vi "Trim Channel Info.vi"(8 "error IO":errorcluster, 11 "Raw Channel Info":string[][](array[string])) -> (0 "error out":errorcluster, 3 "Trimmed Channel Info":T1[](array[typedef]))   [LabVIEW 2021, in "myRIOMetaDataObj.lvclass"]
uses:
  myRIOMetaDataObj.lvclass
  IODetail.ctl
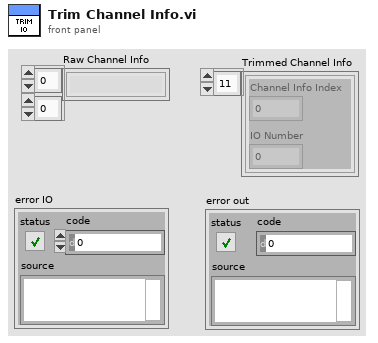
[diagram p1: front panel]
types:
  T1 = typedef "myRIOMetaDataObj.lvclass/IODetail.ctl" = cluster{"Channel Info Index":i8, "IO Number":i8}
  T2 = enum16{"Initial", "Get Channel Info Index by Name", "Get Channel Info by Index", "Get Channel Info by Img Index"}
  T3 = typedef "myRIOMetaDataObj.lvclass/ChannelInfo.ctl" = cluster{"Priority":u16, "Channel Shortcut":string, "Channel Description":string, "Channl Image Index":u16}
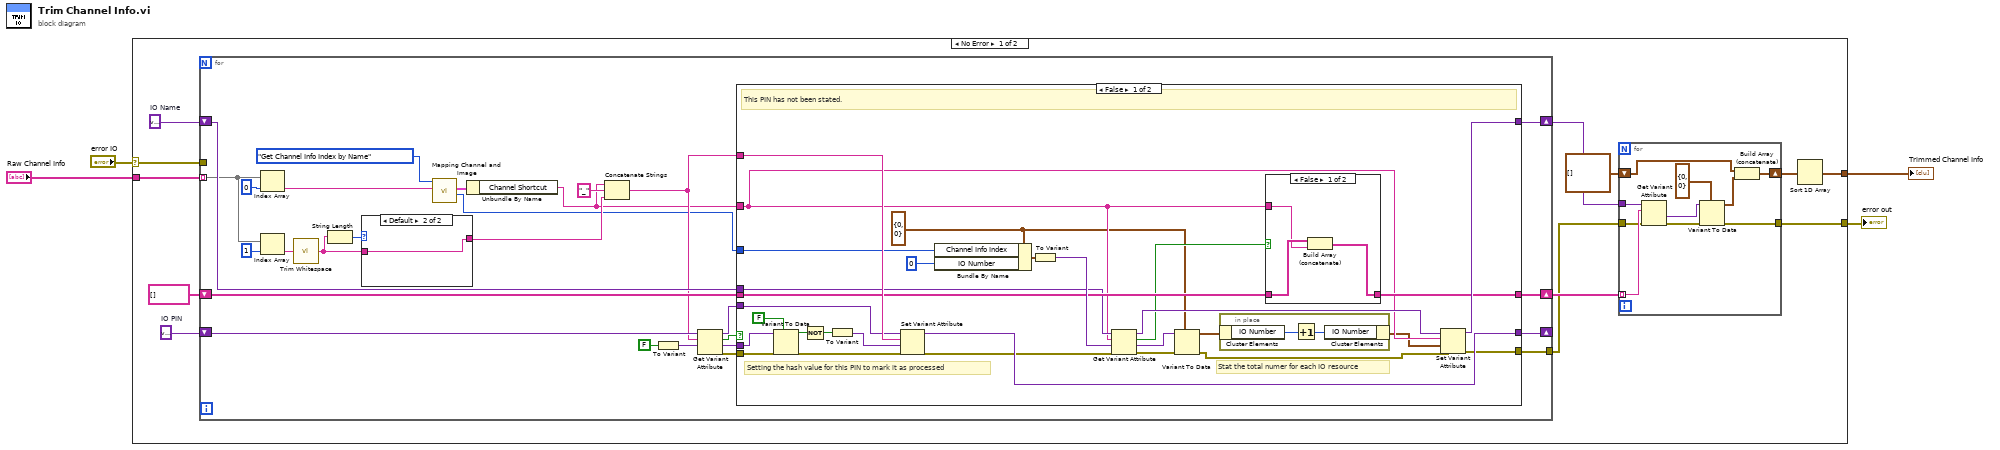
[diagram p0: block diagram]
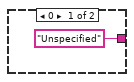
[diagram p2: hidden frame]
diagram:
  n1 = case shown="No Error" "error IO" {
    selector: "error IO" -> [w10 w95]
    tunnel: [w11 w95] -> w4
    tunnel: "Raw Channel Info" -> [w9 _]
    tunnel: [w5 _] -> w1
    frame No Error {
      w8 = variant  # IO PIN
      w16 = variant  # IO Name
      n2 = for {
        tunnel: w9 -> [w36] mode=indexing
        shift-right: [w45] -> w13
        shift-left: w16 -> [w38]
        shift-right: [w39] -> w14
        shift-left: string[] [] -> [w40]
        tunnel: w10 -> [_]
        shift-right: [w44] -> _
        shift-left: w8 -> [w52]
        tunnel: [w28] -> w7
        n3 = Index Array(array=w36, index=0) -> (element=w32:string)
        n4 = Index Array(array=w36, index=1) -> (element=w43:string)
        n5 = call <vilib>:"Trim Whitespace.vi"("string"=w43) -> ("trimmed string"=w41:string)  [unwired: 1 in]
        n6 = String Length(string=w41) -> (length=w42:i32)
        n7 = case shown="Default" w42 {
          tunnel: w41 -> [_ w55]
          tunnel: ["Unspecified" w55] -> w35
          frame 0 {
          }
          frame Default {
          }
        }
        n8 = call "Mapping Channel and Image.vi"("Channel Name"=w32, "Operation"=T2."Get Channel Info Index by Name") -> ("Channel Info Index Out"=w29:u16, "Channel Info"=w31:T3)  [unwired: 8 in]
        n9 = Unbundle By Name(w31) -> ("Channel Shortcut"=w30:string)
        n10 = Concatenate Strings(w30, "_" ("string"), w35) -> (w33:string)
        n11 = To Variant(anything=FALSE) -> (Variant=w51:variant)
        n12 = Get Variant Attribute(Variant=w52, name=w33, default value (empty Variant)=w51) -> (duplicate Variant=w49:variant, found=w50:bool, value=w48:variant, error out=w46:errorcluster)  [unwired: 1 in]
        n13 = case shown="False" w50 {
          tunnel: w49 -> [w79 w94]
          tunnel: w48 -> [w84 _]
          tunnel: w33 -> [w80 _]
          tunnel: w46 -> [w77 w93]
          tunnel: [w76 w92] -> w45
          tunnel: [w75 w94] -> w44
          tunnel: [w74 w93] -> w28
          tunnel: w40 -> [w67 w91]
          tunnel: [w66 w91] -> w39
          tunnel: w38 -> [w64 w92]
          tunnel: w30 -> [w63 _]
          tunnel: w29 -> [w62 _]
          frame False {
            w59 = T1 {"Channel Info Index"=0, "IO Number"=0} ("IO Detail")
            # "Stat the total numer for each IO resource"
            # "Setting the hash value for this PIN to mark it as processed"
            # "This PIN has not been stated."
            n14 = Variant To Data(error in=w77, type=FALSE, Variant=w84) -> (data=w83:bool, error out=w78:errorcluster)
            n15 = Not(x=w83) -> (.not. x?=w82:bool)
            n16 = To Variant(anything=w82) -> (Variant=w81:variant)
            n17 = Set Variant Attribute(Variant=w79, name=w80, value=w81, error in=w78) -> (Variant out=w75:variant, error out=w70:errorcluster)  [unwired: 1 out]
            n18 = Bundle By Name(cluster=w59, "Channel Info Index"=w62, "IO Number"=i8 0) -> (w60:T1)
            n19 = To Variant(anything=w60) -> (Variant=w71:variant)
            n20 = Get Variant Attribute(Variant=w64, name=w63, default value (empty Variant)=w71, error in=w70) -> (duplicate Variant=w72:variant, found=w65:bool, value=w68:variant, error out=w69:errorcluster)
            n21 = Variant To Data(error in=w69, type=w59, Variant=w68) -> (data=w58:T1, error out=w56:errorcluster)
            n22 = in-place {
              n23 = in-place-cluster #1(w58) -> ("IO Number"=w86:i8)
              n24 = Increment(x=w86) -> (x+1=w85:i8)
              n25 = in-place-cluster #1("IO Number"=w85) -> (w57:T1)
            }
            n26 = case shown="False" w65 {
              tunnel: w67 -> [w89 w90]
              tunnel: [w88 w90] -> w66
              tunnel: w63 -> [w87 _]
              frame False {
                n27 = Build Array (concatenate)(w89, w87) -> (w88:string[])
              }
              frame True {
              }
            }
            n28 = Set Variant Attribute(Variant=w72, name=w63, value=w57, error in=w56) -> (Variant out=w76:variant, error out=w74:errorcluster)  [unwired: 1 out]
          }
          frame True {
            # "This PIN needs to be trimmed."
          }
        }
      }
      n29 = for {
        tunnel: w14 -> [w24] mode=indexing
        tunnel: w13 -> [w26]
        shift-right: [w22] -> w6
        shift-left: T1[] [] -> [w20]
        tunnel: [w21] -> w11
        tunnel: w7 -> [w17]
        n30 = Get Variant Attribute(Variant=w26, name=w24, error in=w17) -> (value=w25:variant, error out=w23:errorcluster)  [unwired: 1 in, 2 out]
        n31 = Variant To Data(error in=w23, type=T1 {"Channel Info Index"=0, "IO Number"=0} ("IO Detail"), Variant=w25) -> (data=w18:T1, error out=w21:errorcluster)
        n32 = Build Array (concatenate)(w20, w18) -> (w22:T1[])
      }
      n33 = Sort 1D Array(array=w6) -> (sorted array=w5:T1[])
    }
    frame Error {
    }
  }
  "error out" <- w4
  "Trimmed Channel Info" <- w1
